vi "IniConfig.vi"(6 "产品型号":refnum<vi>, 7 "PassYeild":refnum<vi>, 8 "error in (no error)":errorcluster, 9 "Operate":enum16{"Write", "Read"}(ring), 10 "ModelName":string, 11 "ConfigIn":T1={"TestedNum"=10, "PassedNum"=5, "FailedNum"=5, "Slot1TestedNum"=10, "Slot2TestedNum"=10, "Slot3TestedNum"=10, "Slot4TestedNum"=10, "GuiVer"="1.0", "LimitFileVer"="1.0", "Login Name"="", "Password"="", "SN_Head"="0", "SN_Length"=1, "AbortOnFail"=FALSE, "DataBaseEnable?"=FALSE, "FixtureID"="", "ShowSkipStep?"=FALSE}) -> (0 "error out":errorcluster, 1 "ShowToolBar":bool, 2 "ShowMenu":bool, 3 "ConfigOut":T1={"TestedNum"=10, "PassedNum"=5, "FailedNum"=5, "Slot1TestedNum"=10, "Slot2TestedNum"=10, "Slot3TestedNum"=10, "Slot4TestedNum"=10, "GuiVer"="1.0", "LimitFileVer"="1.0", "Login Name"="", "Password"="", "SN_Head"="0", "SN_Length"=1, "AbortOnFail"=FALSE, "DataBaseEnable?"=FALSE, "FixtureID"="", "ShowSkipStep?"=FALSE}, 4 "Button":bool, 5 "AutoDetPort":bool)   [LabVIEW 2013]
uses:
  SysControl/Setup.ctl
  SourceCode/GlobalValue.vi
  <vilib>/Utility/config.llb/Read Key (U32).vi
  <vilib>/Utility/config.llb/Read Key (String).vi
  <vilib>/Utility/config.llb/Read Key (I32).vi
  <vilib>/Utility/file.llb/Write To Spreadsheet File (DBL).vi
  <vilib>/Utility/config.llb/Write Key (U32).vi
  <vilib>/Utility/config.llb/NI_LVConfig.lvlib
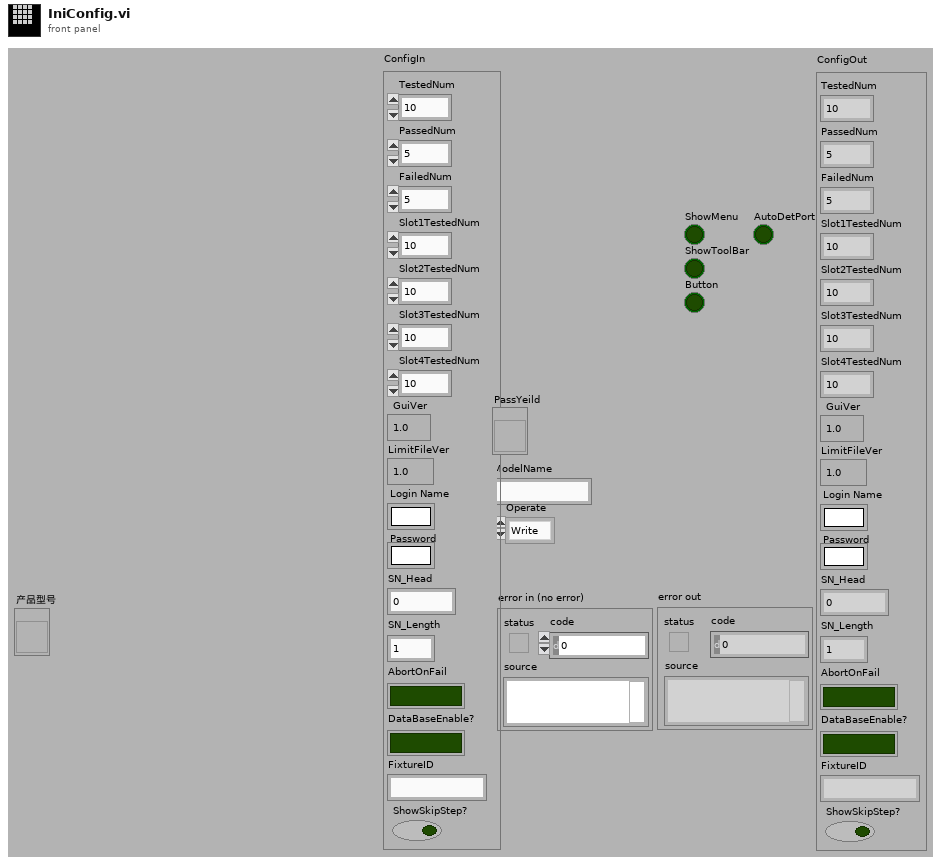
[diagram p1: front panel]
types:
  T1 = typedef "Setup.ctl" = cluster{"TestedNum":u32, "PassedNum":u32, "FailedNum":u32, "Slot1TestedNum":u32, "Slot2TestedNum":u32, "Slot3TestedNum":u32, "Slot4TestedNum":u32, "GuiVer":string, "LimitFileVer":string, "Login Name":string, "Password":string, "SN_Head":string, "SN_Length":i32, "AbortOnFail":bool, "DataBaseEnable?":bool, "FixtureID":string, "ShowSkipStep?":bool}
  T2 = typedef "NI_LVConfig.lvlib/Config Data RefNum.ctl" = refnum<k1>
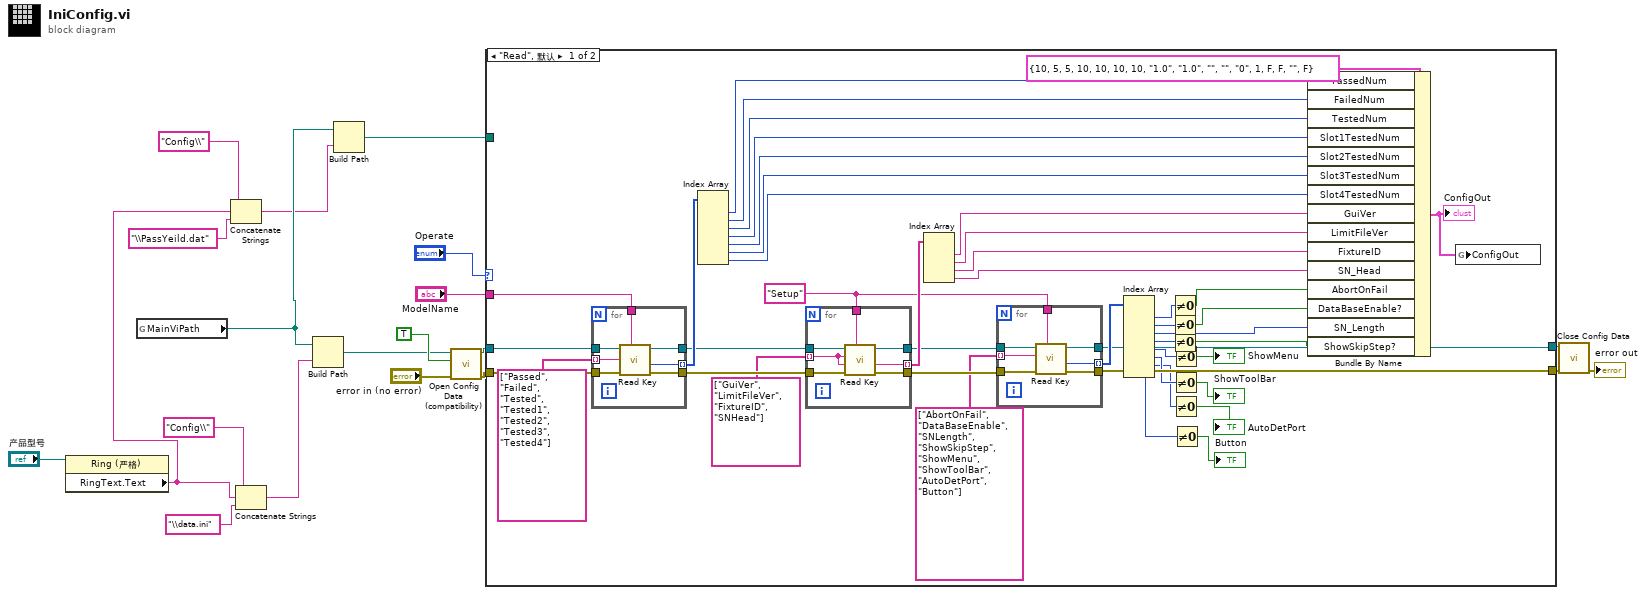
[diagram p0: block diagram]
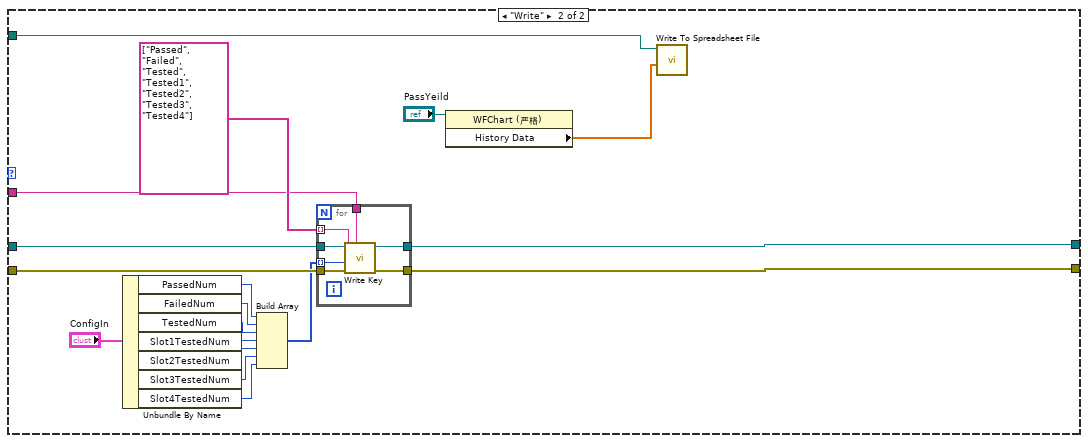
[diagram p2: hidden frame]
diagram:
  n1 = property on="属性节点" class="Ring (严格)"(reference="产品型号") -> ("RingText.Text"=w1:string)  [unwired: 1 in, 2 out]
  n2 = global read "GlobalValue.vi" "MainViPath"() -> (w9:path)
  n3 = Concatenate Strings("Config\\" ("字符串"), w1, "\\PassYeild.dat" ("名称或相对路径")) -> (w2:string)
  n4 = Concatenate Strings("Config\\" ("字符串"), w1, "\\data.ini" ("名称或相对路径")) -> (w5:string)
  n5 = Build Path(base path=w9, name or relative path=w5) -> (appended path=w13:path)
  n6 = Build Path(base path=w9, name or relative path=w2) -> (appended path=w10:path)
  n7 = call <vilib>:"Open Config Data (compatibility).vi"("error in (no error)"="error in (no error)", "create file if necessary (T)"=TRUE, "configuration file path"=w13) -> ("error out"=w18:errorcluster, "refnum"=w19:T2)  [unwired: 6 in, 1 out]
  n8 = case shown="\"Read\", 默认" "Operate" {
    tunnel: w19 -> [w64 w103]
    tunnel: w18 -> [w63 w102]
    tunnel: "ModelName" -> [w42 w100]
    tunnel: [w34 w89] -> w17
    tunnel: [w33 w90] -> w16
    tunnel: w10 -> [_ w87]
    frame "Read", Default {
      w41 = "Setup" ("section")
      n9 = for {
        tunnel: w64 -> [w85]
        tunnel: w63 -> [w84]
        tunnel: [w83] -> w53
        tunnel: [w82] -> w52
        tunnel: w42 -> [w81]
        tunnel: [w80] -> w61 mode=indexing
        tunnel: string[] ["Passed", "Failed", "Tested", "Tested1", "Tested2", "Tested3", "Tested4"] -> [w79] mode=indexing
        n10 = call-poly <vilib>:"Read Key.vi"("section"=w81, "error in (no error)"=w84, "key"=w79, "refnum"=w85) -> ("error out"=w83:errorcluster, "value"=w80:u32, "refnum out"=w82:T2)  [unwired: 1 in, 4 out]
      }
      n11 = Index Array(array=w61) -> (element #1=w60:u32, element #2=w59:u32, element #3=w58:u32, element #4=w57:u32, element #5=w56:u32, element #6=w55:u32, element #7=w54:u32)  [unwired: 7 in]
      n12 = for {
        tunnel: w52 -> [w78]
        tunnel: w53 -> [w77]
        tunnel: [w76] -> w44
        tunnel: [w75] -> w45
        tunnel: w41 -> [w74]
        tunnel: [w73] -> w50 mode=indexing
        tunnel: string[] ["GuiVer", "LimitFileVer", "FixtureID", "SNHead"] -> [w72] mode=indexing
        n13 = call-poly <vilib>:"Read Key.vi"("section"=w74, "error in (no error)"=w77, "default value"=w72, "key"=w72, "refnum"=w78) -> ("error out"=w76:errorcluster, "value"=w73:string, "refnum out"=w75:T2)  [unwired: 1 in, 3 out]
      }
      n14 = Index Array(array=w50) -> (element #1=w49:string, element #2=w48:string, element #3=w47:string, element #4=w46:string)  [unwired: 4 in]
      n15 = for {
        tunnel: w45 -> [w71]
        tunnel: w44 -> [w70]
        tunnel: [w69] -> w33
        tunnel: [w68] -> w34
        tunnel: w41 -> [w67]
        tunnel: [w66] -> w40 mode=indexing
        tunnel: string[] ["AbortOnFail", "DataBaseEnable", "SNLength", "ShowSkipStep", "ShowMenu", "ShowToolBar", "AutoDetPort", "Button"] -> [w65] mode=indexing
        n16 = call-poly <vilib>:"Read Key.vi"("section"=w67, "error in (no error)"=w70, "key"=w65, "refnum"=w71) -> ("error out"=w69:errorcluster, "value"=w66:i32, "refnum out"=w68:T2)  [unwired: 1 in, 4 out]
      }
      n17 = Index Array(array=w40) -> (element #1=w39:i32, element #2=w38:i32, element #3=w37:i32, element #4=w31:i32, element #5=w28:i32, element #6=w26:i32, element #7=w24:i32, element #8=w22:i32)  [unwired: 8 in]
      n18 = Not Equal To 0?(x=w39) -> (x != 0?=w35:bool)
      n19 = Not Equal To 0?(x=w38) -> (x != 0?=w36:bool)
      n20 = Not Equal To 0?(x=w31) -> (x != 0?=w30:bool)
      n21 = Not Equal To 0?(x=w28) -> (x != 0?=→"ShowMenu":bool)
      n22 = Not Equal To 0?(x=w26) -> (x != 0?=→"ShowToolBar":bool)
      n23 = Not Equal To 0?(x=w24) -> (x != 0?=→"AutoDetPort":bool)
      n24 = Not Equal To 0?(x=w22) -> (x != 0?=→"Button":bool)
      n25 = Bundle By Name(cluster=T1 {"TestedNum"=10, "PassedNum"=5, "FailedNum"=5, "Slot1TestedNum"=10, "Slot2TestedNum"=10, "Slot3TestedNum"=10, "Slot4TestedNum"=10, "GuiVer"="1.0", "LimitFileVer"="1.0", "Login Name"="", "Password"="", "SN_Head"="0", "SN_Length"=1, "AbortOnFail"=FALSE, "DataBaseEnable?"=FALSE, "FixtureID"="", "ShowSkipStep?"=FALSE} ("IN 2"), "PassedNum"=w60, "FailedNum"=w59, "TestedNum"=w58, "Slot1TestedNum"=w57, "Slot2TestedNum"=w56, "Slot3TestedNum"=w55, "Slot4TestedNum"=w54, "GuiVer"=w49, "LimitFileVer"=w48, "FixtureID"=w47, "SN_Head"=w46, "AbortOnFail"=w35, "DataBaseEnable?"=w36, "SN_Length"=w37, "ShowSkipStep?"=w30) -> (w29:T1)
      "ConfigOut" <- w29
      n26 = global write "GlobalValue.vi" "ConfigOut"(w29) -> ()
    }
    frame "Write" {
      n27 = Unbundle By Name("ConfigIn") -> ("PassedNum"=w98:u32, "FailedNum"=w97:u32, "TestedNum"=w96:u32, "Slot1TestedNum"=w95:u32, "Slot2TestedNum"=w94:u32, "Slot3TestedNum"=w93:u32, "Slot4TestedNum"=w92:u32)
      n28 = Build Array(w98, w97, w96, w95, w94, w93, w92) -> (w91:u32[])
      n29 = for {
        tunnel: w103 -> [w110]
        tunnel: w102 -> [w109]
        tunnel: [w108] -> w90
        tunnel: [w107] -> w89
        tunnel: w100 -> [w106]
        tunnel: string[] ["Passed", "Failed", "Tested", "Tested1", "Tested2", "Tested3", "Tested4"] -> [w105] mode=indexing
        tunnel: w91 -> [w104] mode=indexing
        n30 = call-poly <vilib>:"Write Key.vi"("section"=w106, "error in (no error)"=w109, "value"=w104, "key"=w105, "refnum"=w110) -> ("error out"=w108:errorcluster, "refnum out"=w107:T2)  [unwired: 4 in, 1 out]
      }
      n31 = property on="属性节点" class="WFChart (严格)"(reference="PassYeild") -> ("History Data"=w88:dbl[])  [unwired: 1 in, 2 out]
      n32 = call-poly <vilib>:"Write To Spreadsheet File.vi"("1D data"=w88, "file path (dialog if empty)"=w87) -> ()  [unwired: 6 in, 1 out]
    }
  }
  n33 = call <vilib>:"Close Config Data.vi"("error in (no error)"=w16, "refnum"=w17) -> ("error out"=→"error out":errorcluster)  [unwired: 1 in, 8 out]
